vi "Configure Trigger Characteristics.vi"(5 "RF Burst Slope (0: Positive)":i32(ring) items=["Positive", "Negative"], 6 "RF Burst Level (-30 dBm)":dbl=-30.0, 7 "Period Timer Source (0: Off)":i32(ring) items=["Off", "External", "RF Burst"], 8 "error in (no error)":errorcluster, 9 "Periodic Timer Offset (0.01 seconds)":dbl=0.01, 10 "Periodic Timer Period (0.01 seconds)":dbl=0.01, 11 "VISA resource name":refnum<visa-resource-name>) -> (0 "error out":errorcluster, 3 "VISA resource name out":refnum<visa-resource-name>)   [LabVIEW 2022 SP3, in "Agilent N934X Series.lvlib"]
doc: "Configure the trigger settings.\n\nNote:\nThis VI is only applicable for N9321C, N9322C, N9323C, N9324C models"
uses:
  <instrlib>/Agilent N934X Series/Agilent N934X Series.lvlib
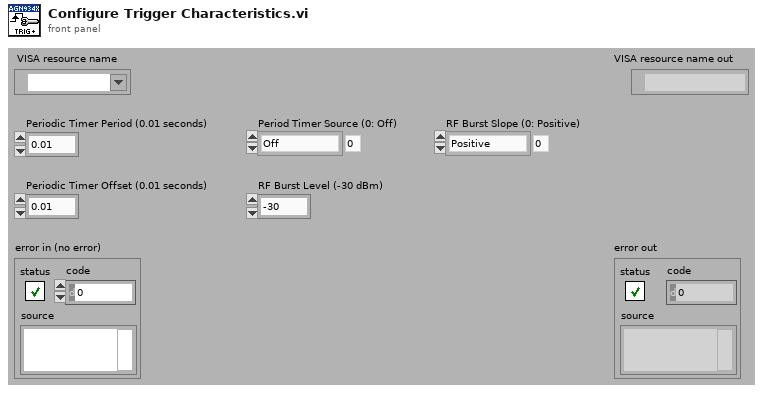
[diagram p1: front panel]
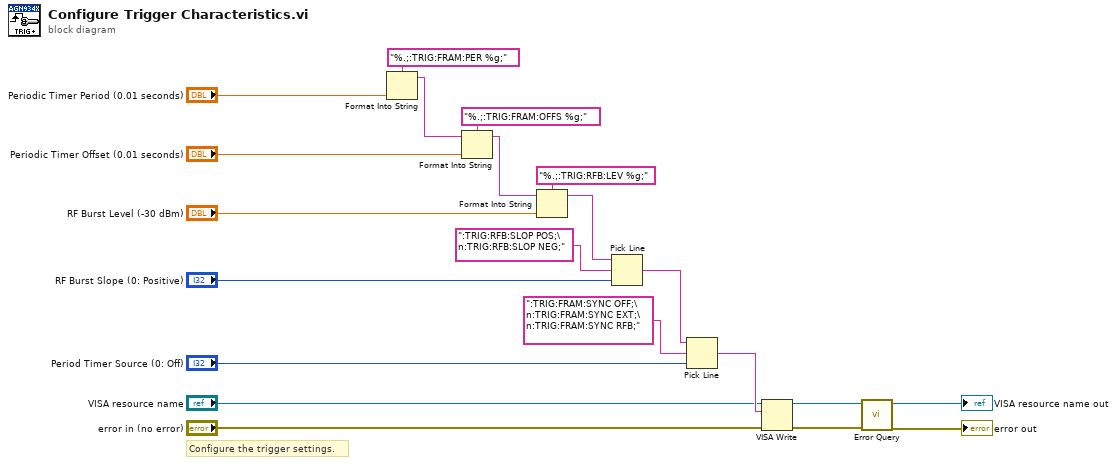
[diagram p0: block diagram]
diagram:
  # "Configure the trigger settings."
  n1 = Format Into String(format string="%.;:TRIG:FRAM:PER %g;", "Periodic Timer Period (0.01 seconds)") -> (resulting string=w19:string)  [unwired: 2 in, 1 out]
  n2 = Format Into String(format string="%.;:TRIG:FRAM:OFFS %g;", initial string=w19, "Periodic Timer Offset (0.01 seconds)") -> (resulting string=w16:string)  [unwired: 1 in, 1 out]
  n3 = Format Into String(format string="%.;:TRIG:RFB:LEV %g;", initial string=w16, "RF Burst Level (-30 dBm)") -> (resulting string=w11:string)  [unwired: 1 in, 1 out]
  n4 = Pick Line(string ("")=w11, multi-line string=":TRIG:RFB:SLOP POS;\n:TRIG:RFB:SLOP NEG;", line index="RF Burst Slope (0: Positive)") -> (output string=w8:string)
  n5 = Pick Line(string ("")=w8, multi-line string=":TRIG:FRAM:SYNC OFF;\n:TRIG:FRAM:SYNC EXT;\n:TRIG:FRAM:SYNC RFB;", line index="Period Timer Source (0: Off)") -> (output string=w7:string)
  n6 = VISA Write(VISA resource name="VISA resource name", write buffer=w7, error in (no error)="error in (no error)") -> (VISA resource name out=w4:refnum<visa-resource-name>, error out=w3:errorcluster)  [unwired: 1 out]
  n7 = call <instrlib>:"Error Query.vi"("error in (no error)"=w3, "VISA resource name"=w4) -> ("error out"=→"error out":errorcluster, "VISA resource name out"=→"VISA resource name out":refnum<visa-resource-name>)  [unwired: 6 in, 2 out]
